vi "UnitTest-TableLogger.vi"   [LabVIEW 2014]
uses:
  TableLogger_Actor/TableLoggerConfig.ctl
  TableLogger_Actor/TableLoggerTypes.ctl
  TableLogger_Actor/TableLoggerBackupConfig.ctl
  TableLogger_Actor/Messages/InsertData_Msg/InsertData Msg.lvclass/InsertData Msg.ctl
  <vilib>/ActorFramework/Message Enqueuer/Message Enqueuer.lvclass/Message Enqueuer.ctl
  <vilib>/ActorFramework/Message Enqueuer/Enqueue.vi
  <vilib>/ActorFramework/Message Priority Queue/Priority Enqueue.vi
  TableLogger_Actor/Messages/InsertData_Msg/InsertData Msg.lvclass
  <vilib>/ActorFramework/Stop Msg/Stop Msg.lvclass
  TableLogger_Actor/TableLogger_Actor/TableLogger_Actor.lvclass
  TableLogger_Actor/TableLogger_Actor.lvlib
panel:
  # "Look at the block diagram for details about this VI"
types:
  T1 = cluster{"Numeric Data":i32, "Float Data":dbl, "String Data":string, "Enum Data":enum16{"Enum Item 1", "Enum Item 2"}, "Array Data":i32[]}
  T2 = cluster{"Test Start Timestamp":timestamp, "Test End Timestamp":timestamp, "Test Jig Location":string, "Location Time Offset":string, "Test Jig ID":string, "Test Jig Fluid":enum16{"Liquid", "Gas"}, "Test Jig Flow":enum16{"Low", "High"}, "Control Board SN":string, "Site Number":i32, "Operator ID":string, "Operation Number":string, "DUT Serial Number":string, "DUT Product Number":string, "DUT Flow Range":i32, "DUT FW Revision":string, "DUT TP1 Offset":dbl, "DUT TP2 Offset":dbl, "DUT Cut Off1":dbl, "DUT Cut Off2":dbl, "PreCal Flow Meas":cluster{"FC Flow Set":dbl, "FM Flow Measure":dbl, "UUT Data":dbl}[], "PostCal Flow Meas":cluster{"FC Flow Set":dbl, "FM Flow Measure":dbl, "UUT Data":dbl}[], "DUT_Coeff":dbl[], "DUT_Flow_Error":dbl[], "Calibration Result":enum16{"Pass", "Fail"}}
  T3 = typedef "TableLogger_Actor.lvlib/TableLoggerConfig.ctl" = cluster{"TableLogger":T4, "DB File Path":path, "DB Backup Config":T5}
  T4 = typedef "TableLogger_Actor.lvlib/TableLoggerTypes.ctl" = enum16{"CSV Logger", "SQLite Logger"}
  T5 = typedef "TableLogger_Actor.lvlib/TableLoggerBackupConfig.ctl" = cluster{"Directory":path, "UTC Time Format":bool, "On Launch":bool, "Interval (Hours)":dbl, "Size Multiples (Bytes)":i32}
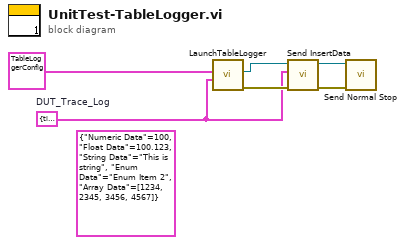
[diagram p0: block diagram]
diagram:
  (unwired) T1 {"Numeric Data"=100, "Float Data"=100.123, "String Data"="This is string", "Enum Data"=enum."Enum Item 2", "Array Data"=[1234, 2345, 3456, 4567]} ("LV Data")
  w1 = T2 {"Test Start Timestamp"=timestamp(0 s since 1904-01-01), "Test End Timestamp"=timestamp(0 s since 1904-01-01), "Test Jig Location"="asdf", "Location Time Offset"="wer", "Test Jig ID"="xcv", "Test Jig Fluid"=enum."Gas", "Test Jig Flow"=enum."High", "Control Board SN"="fgh", "Site Number"=23, "Operator ID"="op", "Operation Number"="op", "DUT Serial Number"="dt", "DUT Product Number"="dt", "DUT Flow Range"=23, "DUT FW Revision"="asdf", "DUT TP1 Offset"=24.0, "DUT TP2 Offset"=546.0, "DUT Cut Off1"=34.0, "DUT Cut Off2"=453.0, "PreCal Flow Meas"=[{"FC Flow Set"=1.0, "FM Flow Measure"=0.0, "UUT Data"=0.0}, {"FC Flow Set"=2.0, "FM Flow Measure"=0.0, "UUT Data"=0.0}, {"FC Flow Set"=3.0, "FM Flow Measure"=0.0, "UUT Data"=0.0}], "PostCal Flow Meas"=[{"FC Flow Set"=1.0, "FM Flow Measure"=0.0, "UUT Data"=0.0}, {"FC Flow Set"=2.0, "FM Flow Measure"=0.0, "UUT Data"=0.0}], "DUT_Coeff"=[1.0, 2.0], "DUT_Flow_Error"=[1.0, 2.0], "Calibration Result"=enum."Fail"}  # DUT_Trace_Log
  n1 = call "LaunchTableLogger.vi"("Data Cluster (for Headers)"=w1, "TableLogger Config"=T3 {"TableLogger"=enum."CSV Logger", "DB File Path"=path "", "DB Backup Config"={"Directory"=path "", "UTC Time Format"=FALSE, "On Launch"=FALSE, "Interval (Hours)"=0.0, "Size Multiples (Bytes)"=0}} ("DB Path")) -> ("error out"=w6:errorcluster, "TableLogger Actor's Enqueuer"=w4:refnum<class "Message Enqueuer.lvclass">)  [unwired: 6 in, 2 out]
  n2 = call "Send InsertData.vi"("error in (no error)"=w6, "Data"=w1, "Message Enqueuer"=w4) -> ("error out"=w5:errorcluster, "Message Enqueuer out"=w3:refnum<class "Message Enqueuer.lvclass">)  [unwired: 7 in]
  n3 = call <vilib>:"Send Normal Stop.vi"("error in (no error)"=w5, "Message Enqueuer"=w3) -> ()  [unwired: 9 in, 1 out]
